vi "TestExec.Configure Test Executive Station Read and Dialog.vi"(9 "Dialog":bool, 11 "TE Config Folder":path=path "C:/MTE/Test Executive/Config") -> (1 "Changed":bool, 3 "Config Out":T1={"Sta App"=path "C:/MTE/Eyetube Calibration/Config/Python/HmdLensController/hmd_tester_python/hmdtester/test_scripts/lens_cal.py", "Station Config"=path "C:/MTE/Eyetube Calibration/Config/Python/new_calib_tree", "ListenPort"=8502, "Sta Name"="", "Station Folder"=path "C:/MTE/Eyetube Calibration/Config/Python/new_calib_tree"})   [LabVIEW 2018]
uses:
  Test Executive/Test Executive/Controls and Type Defs/TestExec.Config Dialog State.ctl
  <vilib>/Utility/config.llb/Read Key (String).vi
  <vilib>/Utility/config.llb/Read Key (U32).vi
  <vilib>/Utility/config.llb/Read Key (Path).vi
  <vilib>/Utility/config.llb/Write Key (String).vi
  <vilib>/Utility/config.llb/Write Key (U32).vi
  <vilib>/Utility/config.llb/Write Key (Path).vi
  <vilib>/KATE/Files/File Utils.lvlib
  <vilib>/Utility/config.llb/NI_LVConfig.lvlib
panel:
  out "Tab Control":enum32{"Inputs", "Data", "Outputs"}(tab)=enum."Data"
  out "Folder Exists":bool caption="Exists"
  in  "Available Applications":u16(ring) items=["Audio Test App.exe", "SoundCheck Data Analysis App.exe", "Base Station.exe", "Base Station OQC Test.exe", "Camera_Calibration App.exe", "Dual_Servo_Controllerexe.exe", "Circle Test App.exe", "Circle Test App.exe", "Circle Test Result Analyzer_V2.exe", "Xlink XML Reader.exe", "Data Warehouse Uploader.exe", "AudioTestUtil.exe", "Function Test App.exe", "FW Load App.exe", "Hmd Control and Status App.exe", "IMU Sensor Calibration Check App.exe", "Lighthouse Console GUI.exe", "Mode Config Utility.exe", "MTE CSV Data File Reader.exe", "Panel Calibration App.exe", "Test Executive.exe", "Tether Cable Test.exe", "Utah Core Audio Test App.exe", "DeleteMe_1502147202_4273_vmpi_service_ui.exe", "vmpi_service.exe", "vmpi_service_install.exe", "vmpi_service_ui.exe", "vmpi_transfer.exe", "WaitAndRestart.exe"]
  in  "Type":enum16{"32 Bit", "64 Bit"}(ring)
  in  "Company":string="Valve"
  in  "Port":u32=8502 caption="Station App Listening Port"
  in  "Station Folder":path=path "C:/MTE/Data/Eyetube Calibration/Capture"
  in  "Station Application":path
  in  "Save":bool
  in  "Cancel":bool
  # "Test Executive ID"
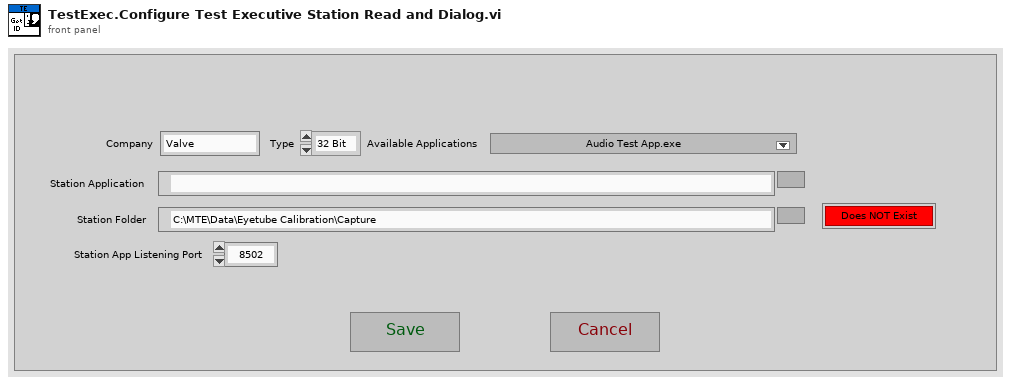
[diagram p1: front panel]
types:
  T1 = cluster{"Sta App":path, "Station Config":path, "ListenPort":u32, "Sta Name":string, "Station Folder":path}
  T2 = typedef "TestExec.Config Dialog State.ctl" = enum16{"Init", "Set Defaults", "Load Config", "Initialize Config", "Initialize Output", "Dialog", "Save", "Update Output", "Done"}
  T3 = enum32{"Invalid", "Standard", "Closed", "Hidden", "Minimized", "Maximized"}
  T4 = typedef "File.Name and Path List Itemctl.ctl" = cluster{"Name":string, "Path":path}
  T5 = cluster{"TE Config Folder":path, "App List":T4[], "TE Config File":path, "State":T2, "Save":bool, "Station Config File":path, "Station Name":string}
  T6 = typedef "NI_LVConfig.lvlib/Config Data RefNum.ctl" = refnum<k1>
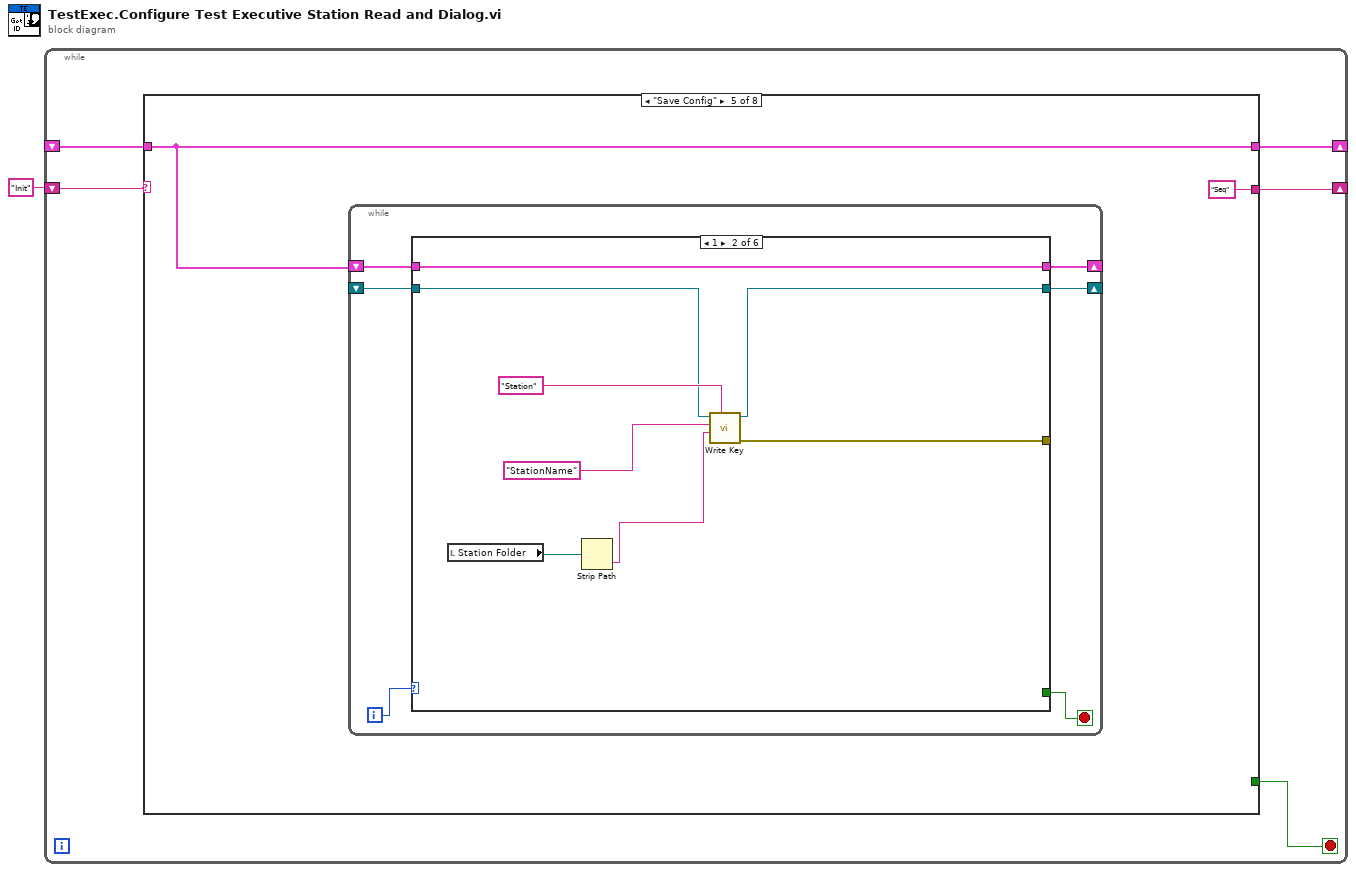
[diagram p0: block diagram]
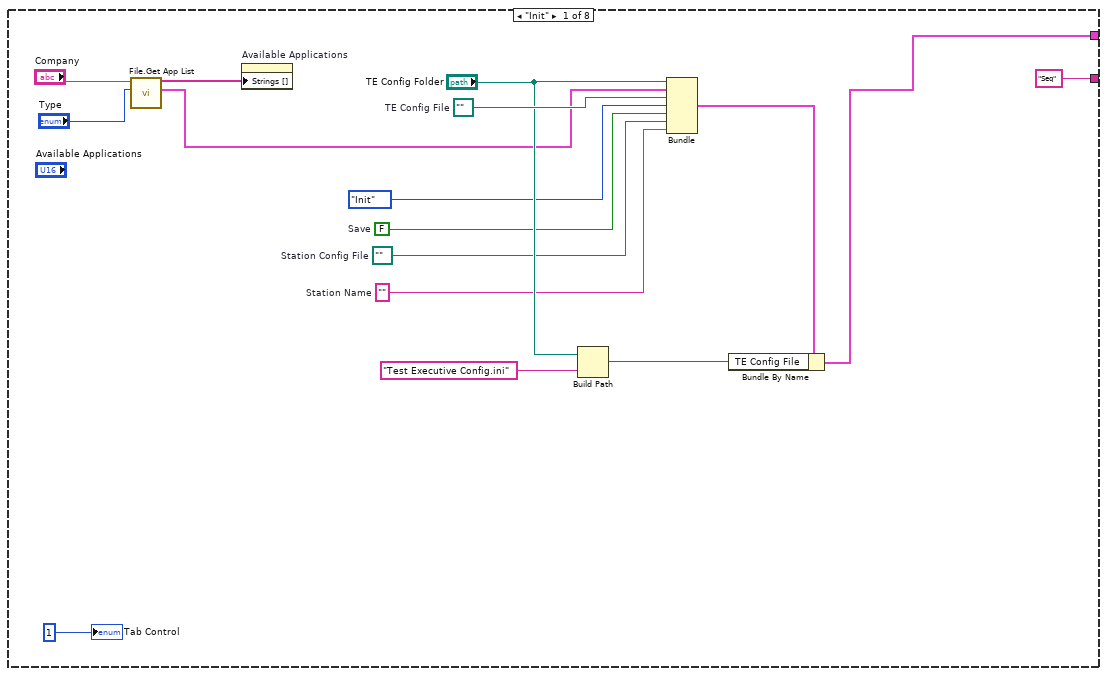
[diagram p2: hidden frame]
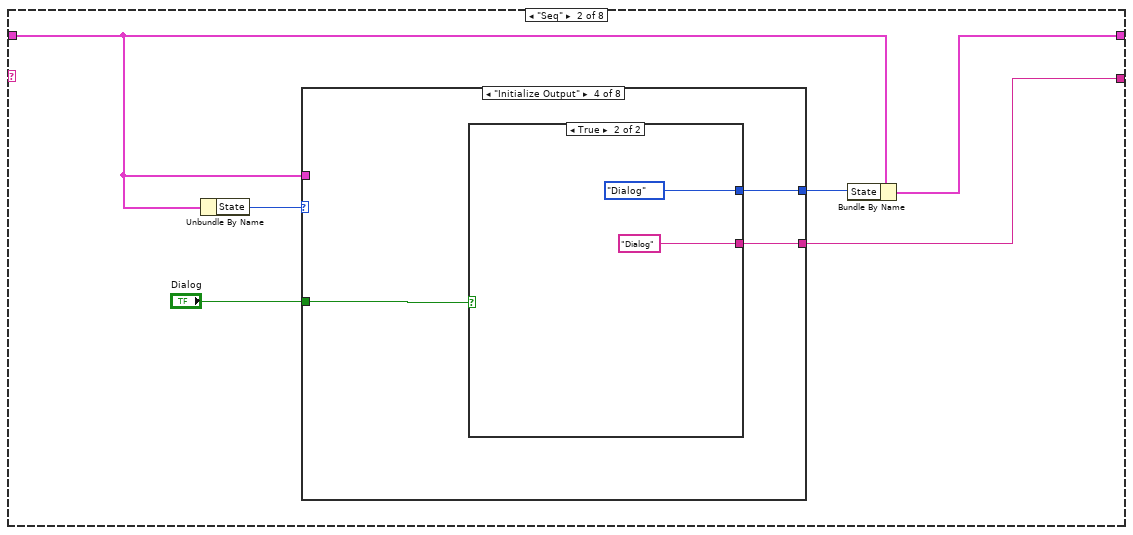
[diagram p3: hidden frame]
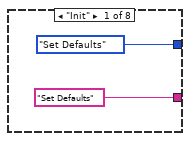
[diagram p4: hidden frame]
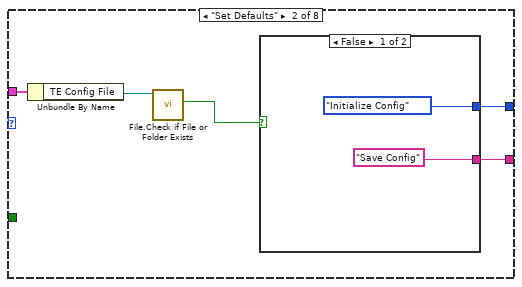
[diagram p5: hidden frame]
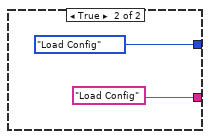
[diagram p6: hidden frame]
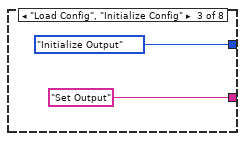
[diagram p7: hidden frame]
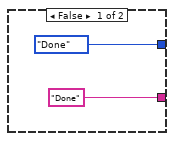
[diagram p8: hidden frame]
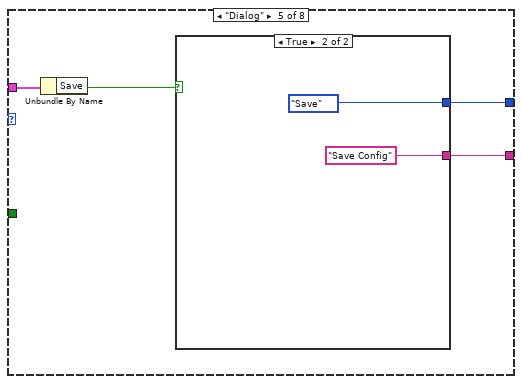
[diagram p9: hidden frame]
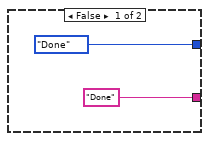
[diagram p10: hidden frame]
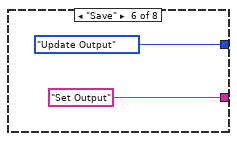
[diagram p11: hidden frame]
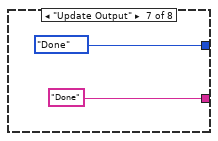
[diagram p12: hidden frame]
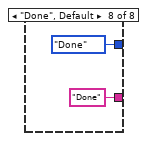
[diagram p13: hidden frame]
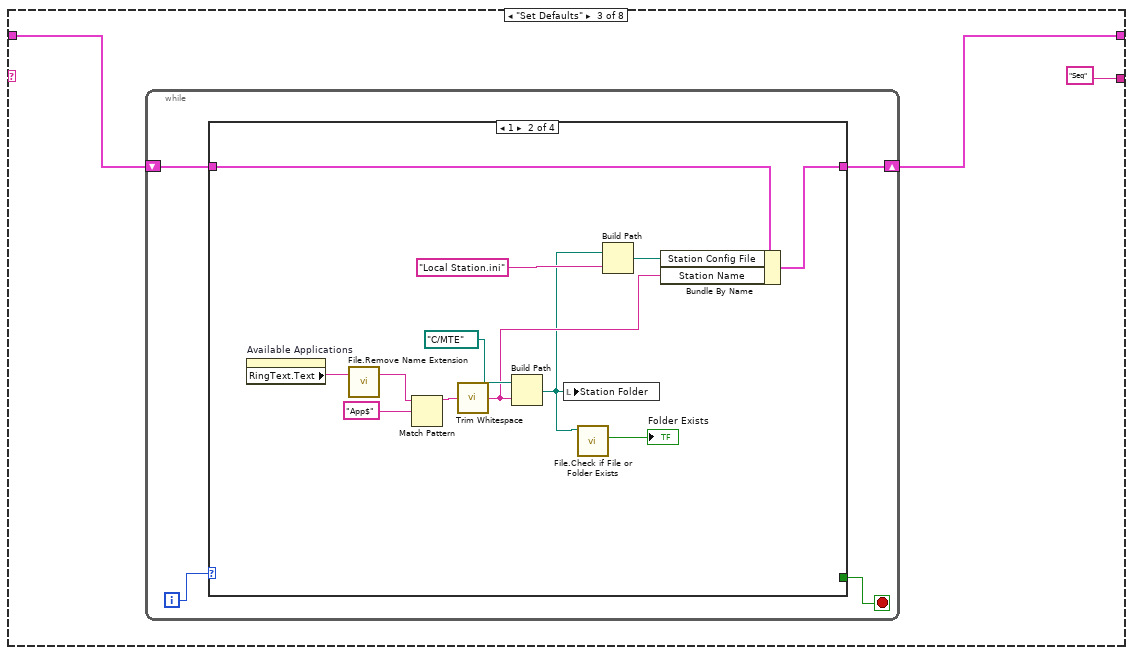
[diagram p14: hidden frame]
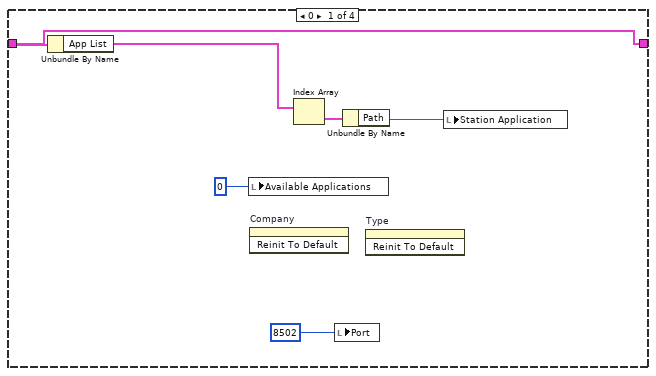
[diagram p15: hidden frame]
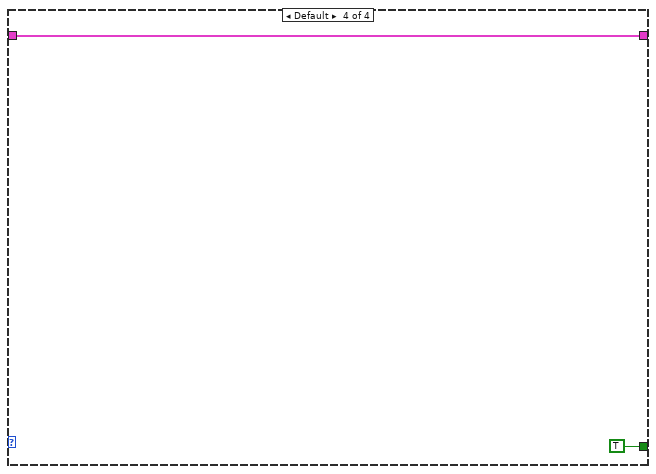
[diagram p17: hidden frame]
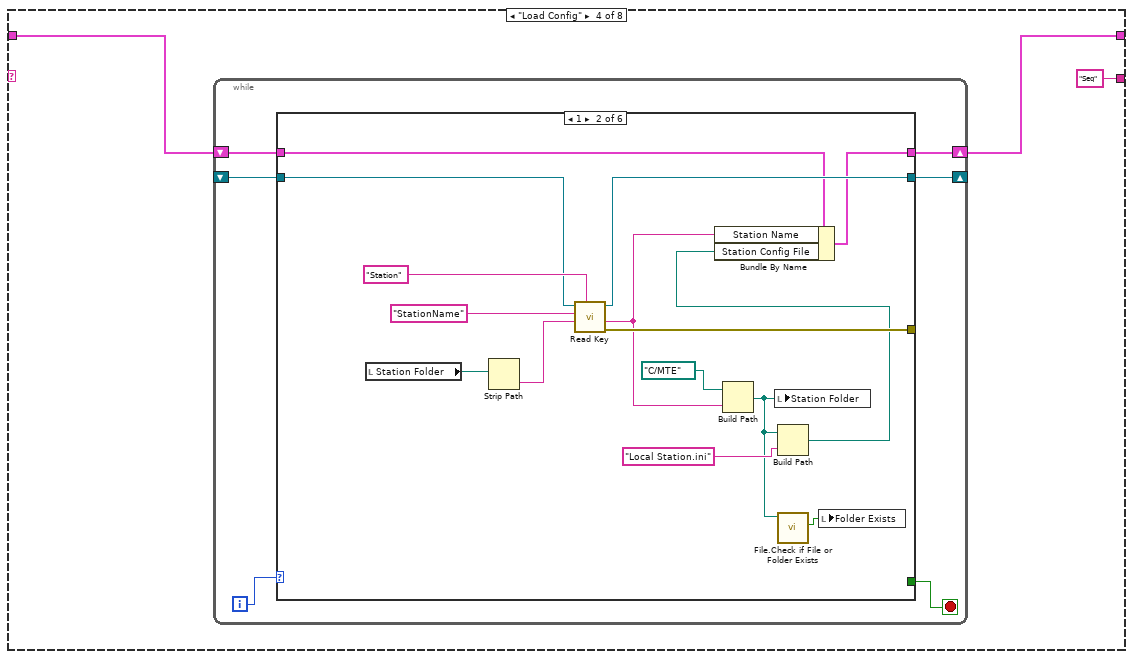
[diagram p18: hidden frame]
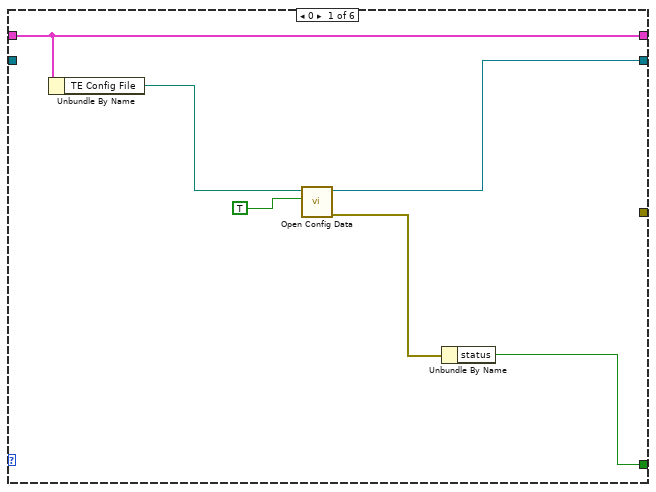
[diagram p19: hidden frame]
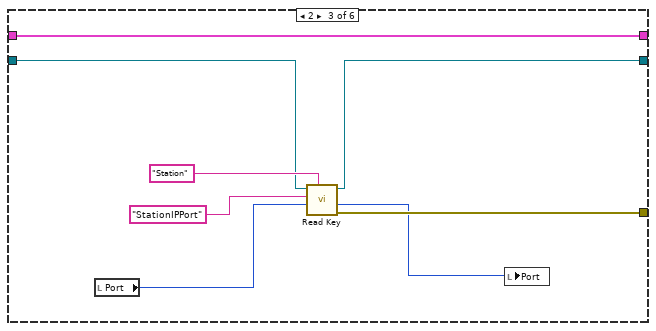
[diagram p20: hidden frame]
diagram:
  n1 = while {
    shift-right: [w4] -> _
    shift-left: _ -> [w6]
    shift-right: [w3] -> _
    shift-left: "Init" -> [w5]
    stop <- w2 stop-if-true
    n2 = case shown="\"Save Config\"" w5 {
      tunnel: w6 -> [_ w26 w64 w92 w156 w200 w234 w244]
      tunnel: [w17 w25 w63 w91 w156 w199 w234 w244] -> w4
      tunnel: ["Seq" w23 "Seq" "Seq" "Seq" "Seq" "Seq" "Done"] -> w3
      tunnel: [_ _ _ _ _ _ _ TRUE] -> w2
      frame "Init" {
        w9 = ""  # Station Name
        w10 = path ""  # Station Config File
        w14 = FALSE  # Save
        w20 = path ""  # TE Config File
        n3 = call "File.Get App List.vi"("Type"="Type", "Prg Folder"="Company") -> ("App List"=w12:T4[], "Available Applications"=w13:string[])  [unwired: 8 in]
        n4 = property on="Available Applications" class="Ring (strict)"("Strings []"=w13) -> ()  [unwired: 2 in, 2 out]
        n5 = Build Path(base path="TE Config Folder", name or relative path="Test Executive Config.ini") -> (appended path=w16:path)
        n6 = Bundle("TE Config Folder"="TE Config Folder", "App List"=w12, "TE Config File"=w20, "State"=TestExec.Config_Dialog_State."Init", "Save"=w14, "Station Config File"=w10, "Station Name"=w9) -> (w18:T5)  [unwired: 1 in]
        n7 = Bundle By Name(cluster=w18, "TE Config File"=w16) -> (w17:T5)
        "Tab Control" <- 1
      }
      frame "Seq" {
        n8 = Unbundle By Name(w26) -> ("State"=w28:T2)
        n9 = case shown="\"Initialize Output\"" w28 {
          tunnel: "Dialog" -> [_ _ _ w44 _ _ _ _]
          tunnel: w26 -> [_ w35 _ _ w50 _ _ _]
          tunnel: [TestExec.Config_Dialog_State."Set Defaults" ("State") w32 TestExec.Config_Dialog_State."Initialize Output" ("State") w43 w52 TestExec.Config_Dialog_State."Update Output" ("State") TestExec.Config_Dialog_State."Done" ("State") TestExec.Config_Dialog_State."Done" ("State")] -> w24
          tunnel: ["Set Defaults" w31 "Set Output" w42 w51 "Set Output" "Done" "Done"] -> w23
          frame "Init" {
          }
          frame "Set Defaults" {
            n10 = Unbundle By Name(w35) -> ("TE Config File"=w34:path)
            n11 = call <vilib>:"File.Check if File or Folder Exists.vi"("Path"=w34) -> ("Exists"=w33:bool)  [unwired: 6 in, 4 out]
            n12 = case shown="False" w33 {
              tunnel: [TestExec.Config_Dialog_State."Initialize Config" ("State") TestExec.Config_Dialog_State."Load Config" ("State")] -> w32
              tunnel: ["Save Config" "Load Config"] -> w31
              frame False {
              }
              frame True {
              }
            }
          }
          frame "Load Config", "Initialize Config" {
          }
          frame "Initialize Output" {
            n13 = case shown="True" w44 {
              tunnel: [TestExec.Config_Dialog_State."Done" ("State") TestExec.Config_Dialog_State."Dialog" ("State")] -> w43
              tunnel: ["Done" "Dialog"] -> w42
              frame False {
              }
              frame True {
              }
            }
          }
          frame "Dialog" {
            n14 = Unbundle By Name(w50) -> ("Save"=w49:bool)
            n15 = case shown="True" w49 {
              tunnel: [TestExec.Config_Dialog_State."Done" ("State") TestExec.Config_Dialog_State."Save" ("State")] -> w52
              tunnel: ["Done" "Save Config"] -> w51
              frame False {
              }
              frame True {
              }
            }
          }
          frame "Save" {
          }
          frame "Update Output" {
          }
          frame "Done", Default {
          }
        }
        n16 = Bundle By Name(cluster=w26, "State"=w24) -> (w25:T5)
      }
      frame "Set Defaults" {
        n17 = while {
          shift-right: [w66] -> w63
          shift-left: w64 -> [w67]
          i -> [w69]
          stop <- w68 stop-if-true
          n18 = case shown="1" w69 {
            tunnel: [_ _ _ TRUE] -> w68
            tunnel: w67 -> [w75 w81 w88 w89]
            tunnel: [w75 w80 w88 w89] -> w66
            frame 0 {
              n19 = Unbundle By Name(w75) -> ("App List"=w73:T4[])
              n20 = local write "Available Applications"(u16 0) -> ()
              n21 = invoke on="Company" class="Str" method="Reinit To Default"() -> ()  [unwired: 3 in, 3 out]
              n22 = Index Array(array=w73) -> (element=w72:T4)  [unwired: 1 in]
              n23 = local write "Port"(u32 8502 ("Listening Port")) -> ()
              n24 = Unbundle By Name(w72) -> ("Path"=w71:path)
              n25 = invoke on="Type" class="Enum (strict)" method="Reinit To Default"() -> ()  [unwired: 3 in, 3 out]
              n26 = local write "Station Application"(w71) -> ()
            }
            frame 1 {
              n27 = property on="Available Applications" class="Ring (strict)"() -> ("RingText.Text"=w86:string)  [unwired: 2 in, 2 out]
              n28 = call <vilib>:"File.Remove Name Extension.vi"("File Name"=w86) -> ("Name Less Ext"=w84:string)  [unwired: 1 in, 1 out]
              n29 = Match Pattern(string=w84, regular expression="App$") -> (before substring=w83:string)  [unwired: 1 in, 3 out]
              n30 = call <vilib>:"Trim Whitespace.vi"("string"=w83) -> ("trimmed string"=w78:string)  [unwired: 1 in]
              n31 = Build Path(base path=path "C:/MTE" ("Capture Data Output Folder"), name or relative path=w78) -> (appended path=w77:path)
              n32 = local write "Station Folder"(w77) -> ()
              n33 = call <vilib>:"File.Check if File or Folder Exists.vi"("Path"=w77) -> ("Exists"=→"Folder Exists":bool)  [unwired: 6 in, 4 out]
              n34 = Build Path(base path=w77, name or relative path="Local Station.ini") -> (appended path=w79:path)
              n35 = Bundle By Name(cluster=w81, "Station Config File"=w79, "Station Name"=w78) -> (w80:T5)
            }
            frame 2 {
            }
            frame Default {
            }
          }
        }
      }
      frame "Load Config" {
        n36 = while {
          shift-right: [w96] -> _
          shift-left: _ -> [w97]
          shift-right: [w95] -> w91
          shift-left: w92 -> [w94]
          i -> [w99]
          stop <- w98 stop-if-true
          n37 = case shown="1" w99 {
            tunnel: [w103 _ _ _ _ TRUE] -> w98
            tunnel: w97 -> [_ w117 w123 w136 w152 w155]
            tunnel: [w105 w116 w122 w135 _ w155] -> w96
            tunnel: [_ w120 w128 w140 w151 _] -> _
            tunnel: [w101 w111 w121 w134 w149 w154] -> w95
            tunnel: w94 -> [w101 w112 w121 w134 w149 w154]
            frame 0 {
              n38 = Unbundle By Name(w101) -> ("TE Config File"=w100:path)
              n39 = call <vilib>:"Open Config Data.vi"("create file if necessary (T)"=TRUE, "configuration file path"=w100) -> ("error out"=w104:errorcluster, "refnum"=w105:T6)  [unwired: 7 in, 1 out]
              n40 = Unbundle By Name(w104) -> ("status"=w103:bool)
            }
            frame 1 {
              n41 = local read "Station Folder"() -> (w115:path)
              n42 = Strip Path(path=w115) -> (name=w114:string)  [unwired: 1 out]
              n43 = call-poly <vilib>:"Read Key.vi"("section"="Station", "default value"=w114, "key"="StationName" ("section"), "refnum"=w117) -> ("error out"=w120:errorcluster, "value"=w110:string, "refnum out"=w116:T6)  [unwired: 4 in, 1 out]
              n44 = Build Path(base path=path "C:/MTE" ("Capture Data Output Folder"), name or relative path=w110) -> (appended path=w106:path)
              n45 = local write "Station Folder"(w106) -> ()
              n46 = Build Path(base path=w106, name or relative path="Local Station.ini") -> (appended path=w108:path)
              n47 = Bundle By Name(cluster=w112, "Station Name"=w110, "Station Config File"=w108) -> (w111:T5)
              n48 = call <vilib>:"File.Check if File or Folder Exists.vi"("Path"=w106) -> ("Exists"=w107:bool)  [unwired: 6 in, 4 out]
              n49 = local write "Folder Exists"(w107) -> ()
            }
            frame 2 {
              n50 = local read "Port"() -> (w125:u32)
              n51 = call-poly <vilib>:"Read Key.vi"("section"="Station", "default value"=w125, "key"="StationIPPort" ("section"), "refnum"=w123) -> ("error out"=w128:errorcluster, "value"=w124:u32, "refnum out"=w122:T6)  [unwired: 4 in, 1 out]
              n52 = local write "Port"(w124) -> ()
            }
            frame 3 {
              n53 = local read "Station Application"() -> (w137:path)
              n54 = Unbundle By Name(w134) -> ("App List"=w133:T4[])
              n55 = call-poly <vilib>:"Read Key.vi"("section"="Station", "default value"=w137, "key"="StationExePath" ("section"), "refnum"=w136) -> ("error out"=w140:errorcluster, "value"=w132:path, "refnum out"=w135:T6)  [unwired: 4 in, 1 out]
              n56 = Strip Path(path=w132) -> (name=w131:string)  [unwired: 1 out]
              n57 = for {
                tunnel: w133 -> [w145] mode=indexing
                tunnel: w131 -> [w148]
                tunnel: [w143] -> w129
                tunnel: [w142] -> w130
                i -> [w143]
                stop <- w142 stop-if-true
                n58 = Unbundle By Name(w145) -> ("Name"=w144:string)
                n59 = To Lower Case(string=w144) -> (all lower case string=w147:string)
                n60 = To Lower Case(string=w148) -> (all lower case string=w146:string)
                n61 = Equal?(x=w146, y=w147) -> (x = y?=w142:bool)
              }
              n62 = local write "Station Application"(w132) -> ()
              n63 = case shown="True" w130 {
                tunnel: w129 -> [_ w141]
                frame False {
                }
                frame True {
                  n64 = local write "Available Applications"(w141) -> ()
                }
              }
            }
            frame 4 {
              n65 = call <vilib>:"Close Config Data.vi"("write file if changed (T)"=TRUE, "refnum"=w152) -> ("error out"=w151:errorcluster)  [unwired: 8 in, 1 out]
            }
            frame Default {
            }
          }
        }
      }
      frame "Save Config" {
        n66 = while {
          shift-right: [w159] -> _
          shift-left: _ -> [w160]
          shift-right: [w158] -> _
          shift-left: w156 -> [w161]
          i -> [w163]
          stop <- w162 stop-if-true
          n67 = case shown="1" w163 {
            tunnel: [w167 _ _ _ _ TRUE] -> w162
            tunnel: w161 -> [w164 w172 w178 w185 w192 w197]
            tunnel: w160 -> [_ w174 w180 w187 w195 w198]
            tunnel: [w169 w173 w179 w186 _ w198] -> w159
            tunnel: [_ w177 w184 w191 w194 _] -> _
            tunnel: [w164 w172 w178 w185 w192 w197] -> w158
            frame 0 {
              n68 = Unbundle By Name(w164) -> ("TE Config File"=w165:path)
              n69 = call <vilib>:"Open Config Data.vi"("create file if necessary (T)"=TRUE, "configuration file path"=w165) -> ("error out"=w168:errorcluster, "refnum"=w169:T6)  [unwired: 7 in, 1 out]
              n70 = Unbundle By Name(w168) -> ("status"=w167:bool)
            }
            frame 1 {
              n71 = local read "Station Folder"() -> (w171:path)
              n72 = Strip Path(path=w171) -> (name=w170:string)  [unwired: 1 out]
              n73 = call-poly <vilib>:"Write Key.vi"("section"="Station", "value"=w170, "key"="StationName" ("section"), "refnum"=w174) -> ("error out"=w177:errorcluster, "refnum out"=w173:T6)  [unwired: 5 in, 1 out]
            }
            frame 2 {
              n74 = local read "Port"() -> (w181:u32)
              n75 = call-poly <vilib>:"Write Key.vi"("section"="Station", "value"=w181, "key"="StationIPPort" ("section"), "refnum"=w180) -> ("error out"=w184:errorcluster, "refnum out"=w179:T6)  [unwired: 5 in, 1 out]
            }
            frame 3 {
              n76 = local read "Station Application"() -> (w188:path)
              n77 = call-poly <vilib>:"Write Key.vi"("section"="Station", "value"=w188, "key"="StationExePath" ("section"), "refnum"=w187) -> ("error out"=w191:errorcluster, "refnum out"=w186:T6)  [unwired: 5 in, 1 out]
            }
            frame 4 {
              n78 = call <vilib>:"Close Config Data.vi"("write file if changed (T)"=TRUE, "refnum"=w195) -> ("error out"=w194:errorcluster)  [unwired: 8 in, 1 out]
            }
            frame Default {
            }
          }
        }
      }
      frame "Dialog" {
        n79 = control-ref of="This VI"() -> (w207:refnum<vi>)
        n80 = invoke class="VI" method="FP.Open"(reference=w207, "Activate"=TRUE ("Activate?"), "State"=T3."Standard") -> (reference out=w204:refnum<vi>, error out=w203:errorcluster)  [unwired: 2 in, 3 out]
        n81 = Close Reference(reference=w204, error in (no error)=w203) -> (error out=w202:errorcluster)
        n82 = while {
          tunnel: w202 -> [_]
          shift-right: [w208] -> w199
          shift-left: w200 -> [w209]
          stop <- w210 stop-if-true
          n83 = event shown="[1] \"Available Applications\": Value Change" {
            selector: _ -> [_ _]
            dyn-events: _ -> [_ _]
            timeout: _ -> [_ _]
            tunnel: [TRUE _] -> w210
            tunnel: w209 -> [w212 w221]
            tunnel: [w211 w220] -> w208
            event "Cancel", "Save": Value Change; Panel Close {
              n84 = event-data() -> ()  [unwired: 1 in, 3 out]
              n85 = Bundle By Name(cluster=w212, "Save"="Save") -> (w211:T5)
            }
            event "Available Applications": Value Change {
              n86 = event-data() -> ()  [unwired: 1 in, 6 out]
              n87 = Unbundle By Name(w221) -> ("App List"=w225:T4[])
              n88 = property on="Available Applications" class="Ring (strict)"() -> ("RingText.Text"=w230:string, "Value"=w224:u16)  [unwired: 2 in, 2 out]
              n89 = Index Array(array=w225, index=w224) -> (element=w223:T4)
              n90 = call <vilib>:"File.Remove Name Extension.vi"("File Name"=w230) -> ("Name Less Ext"=w229:string)  [unwired: 1 in, 1 out]
              n91 = Unbundle By Name(w223) -> ("Path"=w222:path)
              n92 = local write "Station Application"(w222) -> ()
              n93 = Match Pattern(string=w229, regular expression="App$") -> (before substring=w228:string)  [unwired: 1 in, 3 out]
              n94 = call <vilib>:"Trim Whitespace.vi"("string"=w228) -> ("trimmed string"=w219:string)  [unwired: 1 in]
              n95 = Build Path(base path=path "C:/MTE" ("Capture Data Output Folder"), name or relative path=w219) -> (appended path=w215:path)
              n96 = call <vilib>:"File.Check if File or Folder Exists.vi"("Path"=w215) -> ("Exists"=w216:bool)  [unwired: 6 in, 4 out]
              n97 = local write "Folder Exists"(w216) -> ()
              n98 = local write "Station Folder"(w215) -> ()
              n99 = Build Path(base path=w215, name or relative path="Local Station.ini") -> (appended path=w217:path)
              n100 = Bundle By Name(cluster=w221, "Station Config File"=w217, "Station Name"=w219) -> (w220:T5)
            }
          }
        }
      }
      frame "Set Output" {
        n101 = Unbundle By Name(w234) -> ("Station Name"=w233:string, "Station Config File"=w232:path)
        n102 = local read "Config Out"() -> (w238:T1)
        n103 = Bundle By Name(cluster=w238, "Sta App"="Station Application", "Sta Name"=w233, "Station Folder"="Station Folder", "Station Config"=w232, "ListenPort"="Port") -> (→"Config Out":T1)
      }
      frame "Done", Default {
        w241 = TRUE  # Normal(T)/Debug(F)
        n104 = Unbundle By Name(w244) -> ("Save"=→"Changed":bool)
        n105 = local read "Dialog"() -> (w242:bool)
        n106 = And(x=w242, y=w241) -> (x .and. y?=w240:bool)
        n107 = case shown="True" w240 {
          tunnel: [_ w247] -> _
          frame False {
          }
          frame True {
            n108 = control-ref of="This VI"() -> (w250:refnum<vi>)
            n109 = invoke class="VI" method="FP.Close"(reference=w250) -> (reference out=w249:refnum<vi>, error out=w248:errorcluster)  [unwired: 2 in, 1 out]
            n110 = Close Reference(reference=w249, error in (no error)=w248) -> (error out=w247:errorcluster)
          }
        }
      }
    }
  }
